vi "Save Report Information.vi"(8 "error in (no error)":errorcluster, 10 "Report Information.lvclass":refnum<class "Report Information.lvclass">, 11 "Formatter in":refnum<class "Formatter.lvclass">) -> (0 "error out":errorcluster, 3 "Formatter out":refnum<class "Formatter.lvclass">)   [LabVIEW 2015, in "Formatter.lvclass"]
doc: "This VI will take the Report Information, format it and write it to the permanent report."
uses:
  Formatter.lvclass
  Report Information/Report Information.lvclass
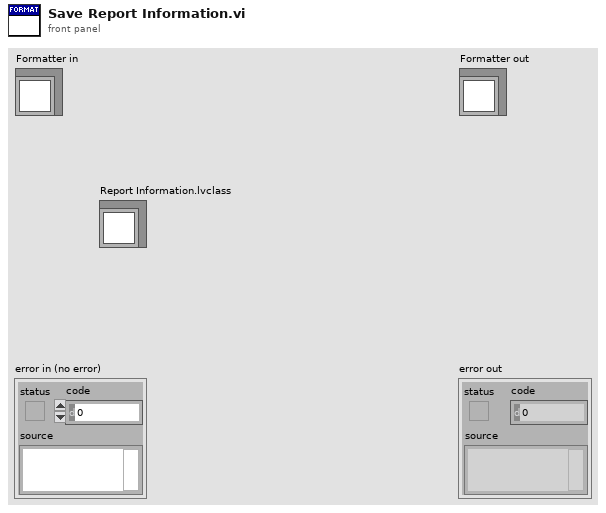
[diagram p1: front panel]
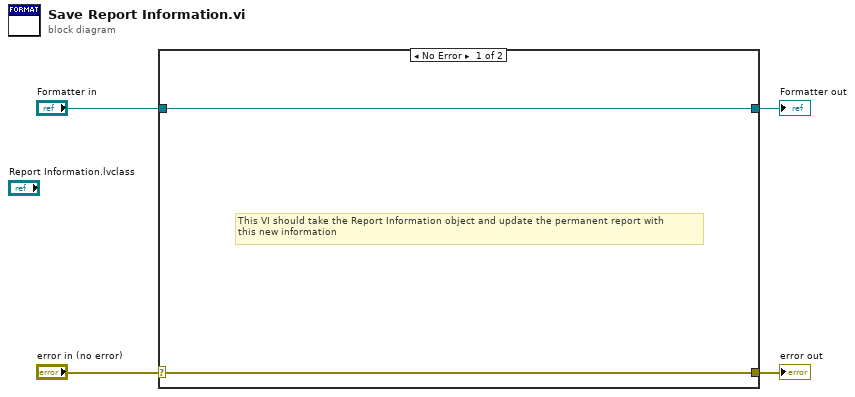
[diagram p0: block diagram]
diagram:
  n1 = case shown="No Error" "error in (no error)" {
    selector: "error in (no error)" -> [w5 w8]
    tunnel: [w5 w8] -> w3
    tunnel: [w6 w7] -> w1
    tunnel: "Formatter in" -> [w6 w7]
    frame No Error {
      # "This VI should take the Report Information object and update the permanent report with\nthis new information"
    }
    frame Error {
    }
  }
  "error out" <- w3
  "Formatter out" <- w1
